vi "macro_vecBuilder5x1FIll.vi"   [LabVIEW 2019, in "Trajectory_Library.lvlib"]
uses:
  MatBuilder_Create.vi
  Trajectory_Library.lvlib
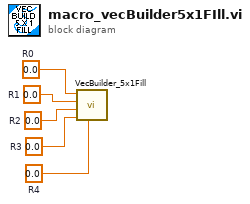
[diagram p0: block diagram]
diagram:
  w1 = 0.0  # R4
  w2 = 0.0  # R3
  w3 = 0.0  # R2
  w4 = 0.0  # R1
  w5 = 0.0  # R0
  n1 = call "VecBuilder_5x1Fill.vi"("R4"=w1, "R3"=w2, "R2"=w3, "R1"=w4, "R0"=w5) -> ()  [unwired: 6 in, 1 out]
